vi "Convert From Celsius.vi"(3 "Temp In":dbl format="%#_13g", 4 "Temp Units":T1) -> (5 "Temp Out":dbl format="%#_13g")   [LabVIEW 2024, in "_Thermal Process Controller.lvclass"]
uses:
  _Thermal Process Controller.lvclass
  Controls/Temperature Units--Enum.ctl
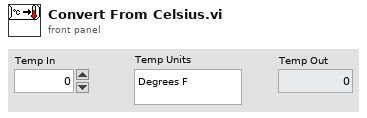
[diagram p1: front panel]
types:
  T1 = typedef "_Thermal Process Controller.lvclass/Temperature Units--Enum.ctl" = enum16{"Degrees F", "Degrees C", "Degrees K"}
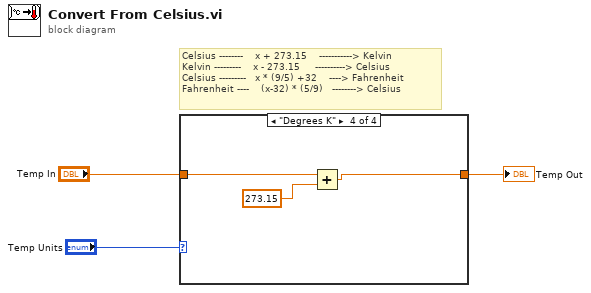
[diagram p0: block diagram]
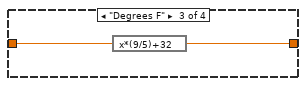
[diagram p4: hidden frame]
diagram:
  # "Celsius --------    x + 273.15    -----------> Kelvin\nKelvin ---------    x - 273.15     ----------> Celsius\nCelsius ---------   x * (9/5) +32    ----> Fahrenheit\nFahrenheit ----    (x-32) * (5/9)   --------> Celsius"
  n1 = case shown="\"Degrees K\"" "Temp Units" {
    tunnel: "Temp In" -> [w4 w5 w7 w10]
    tunnel: [w4 w5 w6 w8] -> w1
    frame Default {
    }
    frame "Degrees C" {
    }
    frame "Degrees F" {
      n2 = expression code="x*(9/5)+32"(w7) -> (w6:dbl)
    }
    frame "Degrees K" {
      n3 = Add(x=w10, y=273.15) -> (x+y=w8:dbl)
    }
  }
  "Temp Out" <- w1
